vi "loadPMData.vi"   [LabVIEW 2012]
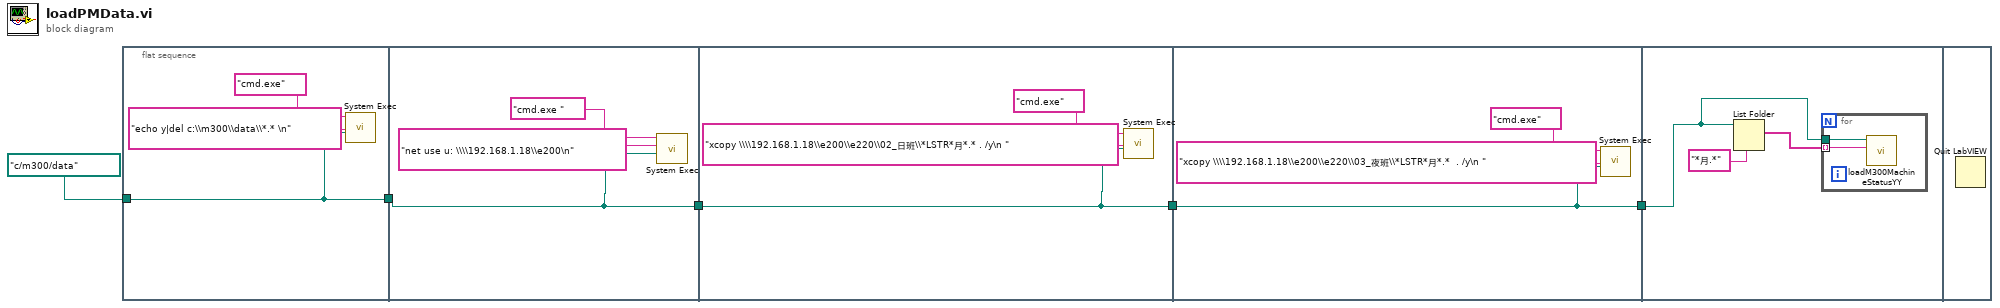
[diagram p0: block diagram]
diagram:
  n1 = flat-sequence {
    tunnel: [w6] -> w2
    tunnel: path "c:/m300/data" ("working directory") -> [w6]
    tunnel: [w9] -> w5
    tunnel: w2 -> [w9]
    tunnel: w5 -> [w12]
    tunnel: [w12] -> w4
    tunnel: w4 -> [w15]
    tunnel: [w15] -> w3
    tunnel: w3 -> [w18]
    frame #0 {
      n2 = call <vilib>:"System Exec.vi"("working directory"=w6, "standard input"="echo y|del c:\\m300\\data\\*.* \n", "command line"="cmd.exe") -> ()  [unwired: 5 in, 4 out]
    }
    frame #1 {
      n3 = call <vilib>:"System Exec.vi"("working directory"=w9, "standard input"="net use u: \\\\192.168.1.18\\e200\n", "command line"="cmd.exe ") -> ()  [unwired: 5 in, 4 out]
    }
    frame #2 {
      n4 = call <vilib>:"System Exec.vi"("working directory"=w12, "standard input"="xcopy \\\\192.168.1.18\\e200\\e220\\02_日班\\*LSTR*月*.* . /y\n ", "command line"="cmd.exe") -> ()  [unwired: 5 in, 4 out]
    }
    frame #3 {
      n5 = call <vilib>:"System Exec.vi"("working directory"=w15, "standard input"="xcopy \\\\192.168.1.18\\e200\\e220\\03_夜班\\*LSTR*月*.*  . /y\n ", "command line"="cmd.exe") -> ()  [unwired: 5 in, 4 out]
    }
    frame #4 {
      n6 = List Folder(path=w18, pattern="*月.*") -> (filenames=w19:string[])  [unwired: 2 in, 3 out]
      n7 = for {
        tunnel: w19 -> [w22] mode=indexing
        tunnel: w18 -> [w21]
        n8 = call "loadM300MachineStatusYY.vi"("name or relative path"=w22, "template (empty)"=w21) -> ()  [unwired: 10 in]
      }
    }
    frame #5 {
      n9 = Quit LabVIEW() -> ()  [unwired: 1 in]
    }
  }
